vi "Query Limit Test Data.vi"(8 "error in (no error)":errorcluster, 9 "Function (0: Volts)":u16(ring) items=["Volts", "Current", "Resistance"], 10 "Test Number (2)":u16=2, 11 "VISA resource name":refnum<visa-resource-name>) -> (0 "error out":errorcluster, 1 "Test Results":string, 2 "Test Passed":bool, 3 "VISA resource name out":refnum<visa-resource-name>)   [LabVIEW 2020, in "Keithley 2450.lvlib"]
doc: "Queries the results of a limit test.\n\n<B>Note:</B> Using this VI will overwrite all triggering settings with settings for a single point taken immediately. For control over the trigger, use the Low Level API."
uses:
  <instrlib>/Keithley 2450/Keithley 2450.lvlib
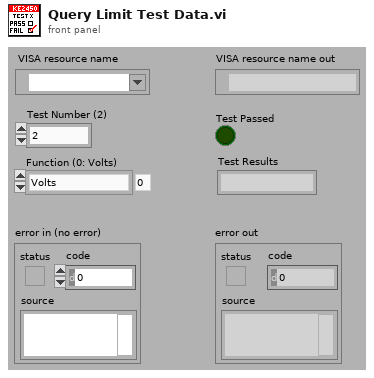
[diagram p1: front panel]
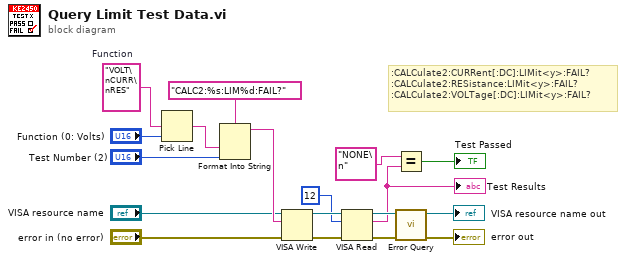
[diagram p0: block diagram]
diagram:
  w5 = "VOLT\nCURR\nRES"  # Function
  # ":CALCulate2:CURRent[:DC]:LIMit<y>:FAIL?\n:CALCulate2:RESistance:LIMit<y>:FAIL?\n:CALCulate2:VOLTage[:DC]:LIMit<y>:FAIL?"
  n1 = Pick Line(multi-line string=w5, line index="Function (0: Volts)") -> (output string=w3:string)  [unwired: 1 out]
  n2 = Format Into String(format string="CALC2:%s:LIM%d:FAIL?", w3, "Test Number (2)") -> (resulting string=w14:string)  [unwired: 2 in, 1 out]
  n3 = VISA Write(VISA resource name="VISA resource name", write buffer=w14, error in (no error)="error in (no error)") -> (VISA resource name out=w10:refnum<visa-resource-name>, error out=w11:errorcluster)  [unwired: 1 out]
  n4 = VISA Read(VISA resource name=w10, byte count=u32 12, error in (no error)=w11) -> (VISA resource name out=w9:refnum<visa-resource-name>, read buffer=w2:string, error out=w8:errorcluster)  [unwired: 1 out]
  "Test Results" <- w2
  n5 = Equal?(x="NONE\n", y=w2) -> (x = y?=→"Test Passed":bool)
  n6 = call <instrlib>:"Error Query.vi"("error in (no error)"=w8, "VISA resource name"=w9) -> ("error out"=→"error out":errorcluster, "VISA resource name out"=→"VISA resource name out":refnum<visa-resource-name>)  [unwired: 8 out]
